vi "Renew TDC Manager.vi"(8 "error in":errorcluster, 9 "TDCManagerRefnum":T1, 10 "TDCManager":T2, 11 "Keep old manager?":bool) -> (0 "error out":errorcluster, 3 "TDCManager out":T2)   [LabVIEW 2016]
uses:
  HPTDC Driver Library Folder/Library files/Typedefs/TDCManager.ctl
  C:/Users/CRT Controller/CRTC Labview Application/Source/HPTDC Driver Library Folder/Library files/hptdc_net4_3.7.0_x64.dll
  HPTDC Driver Library Folder/Library files/hptdc_net4_3.7.0_x64.dll
  HPTDC Driver Library Folder/Library files/Typedefs/TDCManagerRefnum.ctl
  HPTDC Driver Library Folder/HPTDC Driver Library.lvlib
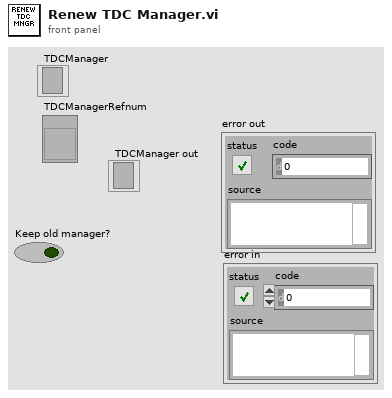
[diagram p1: front panel]
types:
  T1 = typedef "TDCManagerRefnum.ctl" = refnum<vi>
  T2 = typedef "HPTDC Driver Library.lvlib/TDCManager.ctl" = refnum<k24>
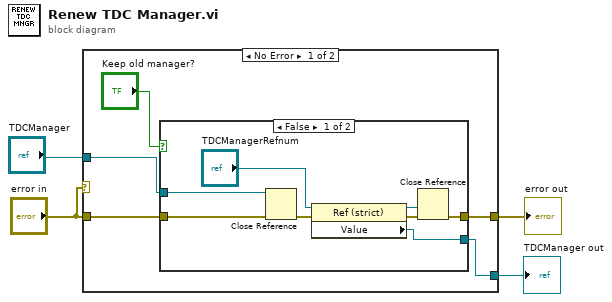
[diagram p0: block diagram]
diagram:
  n1 = case shown="No Error" "error in" {
    tunnel: "TDCManager" -> [w9 w21]
    tunnel: [w7 w20] -> w3
    tunnel: "error in" -> [w6 w20]
    tunnel: [w5 w21] -> w2
    frame No Error {
      n2 = case shown="False" "Keep old manager?" {
        tunnel: w9 -> [w17 w18]
        tunnel: [w16 w19] -> w7
        tunnel: w6 -> [w15 w19]
        tunnel: [w12 w18] -> w5
        frame False {
          n3 = Close Reference(reference=w17, error in (no error)=w15) -> (error out=w10:errorcluster)
          n4 = property class="Ref (strict)"(reference="TDCManagerRefnum", error in=w10) -> (reference out=w14:T1, error out=w13:errorcluster, "Value"=w12:refnum<k24>)
          n5 = Close Reference(reference=w14, error in (no error)=w13) -> (error out=w16:errorcluster)
        }
        frame True {
        }
      }
    }
    frame Error {
    }
  }
  "TDCManager out" <- w2
  "error out" <- w3
